vi "Test PDF Catalog.vi"() -> ()   [LabVIEW 2015]
uses:
  <vilib>/Analysis/NI_AALBase.lvlib
panel:
  in  "Cols":i32=3
  in  "Rows":i32=2
  in  "PDF Path":path=path "C:/Users/hancock/Desktop/test.pdf"
  out "Graph":dbl[](graph)
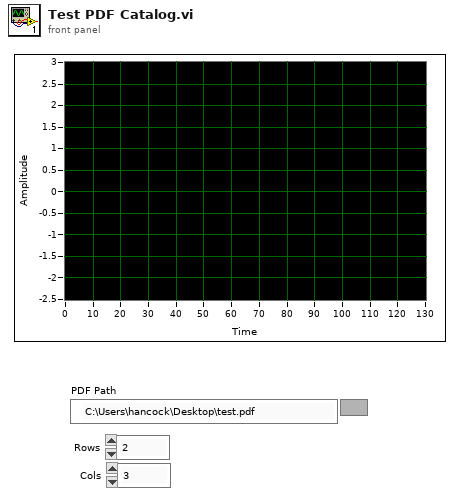
[diagram p1: front panel]
types:
  T1 = typedef "PDF-Catalog.ctl" = cluster{"report":refnum<class "PDF Report Class.lvclass">, "rows":i32, "cols":i32, "border":dbl, "width":dbl, "height":dbl, "next":i32}
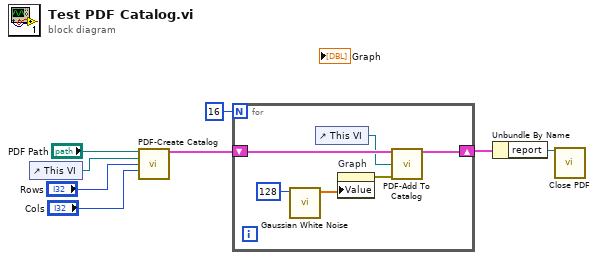
[diagram p0: block diagram]
diagram:
  n1 = control-ref of="This VI"() -> (w7:refnum<vi>)
  n2 = call "PDF-Create Catalog.vi"("PDF Path"="PDF Path", "VI"=w7, "Rows"="Rows", "Cols"="Cols") -> ("catalog"=w6:T1)  [unwired: 10 in, 1 out]
  n3 = for {
    N: 16 -> [_]
    shift-right: [w10] -> w2
    shift-left: w6 -> [w14]
    n4 = call <vilib>:"Gaussian White Noise.vi"("samples"=128) -> ("Gaussian noise pattern"=w12:dbl[])  [unwired: 9 in, 1 out]
    n5 = control-ref of="This VI"() -> (w9:refnum<vi>)
    n6 = property on="Graph" class="WFGraph (strict)"("Value"=w12) -> (error out=w13:errorcluster)  [unwired: 2 in, 1 out]
    n7 = call "PDF-Add To Catalog.vi"("catalog in"=w14, "VI reference"=w9, "error in (no error)"=w13) -> ("catalog out"=w10:T1)  [unwired: 11 in, 1 out]
  }
  n8 = Unbundle By Name(w2) -> ("report"=w3:refnum<class "PDF Report Class.lvclass">)
  n9 = call <vilib>:"Close PDF.vi"("PDF Report"=w3) -> ()  [unwired: 13 in, 2 out]
